vi "Z210 ROUTINE Lister.vi"(0 "unitData in":T3={"typeDevice"=10, "numberDSP"=0}, 2 "DAC#":i32, 3 "buffersParams":T2 {"bufferSize DAC" format="%x"; "bufferAddr DAC" format="%x"; "bufferSize ADC" format="%x"; "bufferAddr ADC" format="%x"}, 5 "error in (no error)":errorcluster, 6 "handicap":dbl=1.0, 7 "Delay Time, ms (100)":i32=-1, 8 "Points":i32, 10 "Linear Correction ADC":T1=[{"scale"=1.0, "offset"=0.0}, {"scale"=1.0, "offset"=0.0}, {"scale"=1.0, "offset"=0.0}, {"scale"=1.0, "offset"=0.0}, {"scale"=1.0, "offset"=0.0}, {"scale"=1.0, "offset"=0.0}, {"scale"=1.0, "offset"=0.0}, {"scale"=1.0, "offset"=0.0}, {"scale"=1.0, "offset"=0.0}, {"scale"=1.0, "offset"=0.0}, {"scale"=1.0, "offset"=0.0}, {"scale"=1.0, "offset"=0.0}, {"scale"=1.0, "offset"=0.0}, {"scale"=1.0, "offset"=0.0}, {"scale"=1.0, "offset"=0.0}, {"scale"=1.0, "offset"=0.0}]) -> (11 "Array":dbl[unit][][](array[numeric]), 14 "unitData out":T3={"typeDevice"=10, "numberDSP"=0}, 17 "buffersParams out":T2 {"bufferSize DAC" format="%x"; "bufferAddr DAC" format="%x"; "bufferSize ADC" format="%x"; "bufferAddr ADC" format="%x"}, 19 "error out":errorcluster)   [LabVIEW 2009]
doc: "Проводится серия следующих измерений: на указанном канале ЦАП устанавливается напряжение в диапазоне 0 - 2,5В (на другом канале ЦАП 0 вольт), затем записываются показания всех каналов АЦП и, если было указано, опрашивается пользователь. Введенное пользователем записывается отдельным каналом в конец.\n\n• unitData — тип устройства и номер сигнального процессора (см. DRIVER Open).\n• AorD — АЦП/ЦАП.\n• numberChannel — номер канала (0 - 16).\n• freq — значение частоты дискретизации в Гц,\n• buffersParams — адреса и размеры буферов данных АЦП и ЦАП в ОЗУ ПК.\n• error in — кластер ошибки. Используется для организации потока данных.\n\n° unitData — тип устройства и номер сигнального процессора (см. DRIVER Open).\n° buffersParams — адреса и размеры буферов данных АЦП и ЦАП в ОЗУ ПК.\n° error out — кластер ошибки. Используется для организации потока данных."
uses:
  Z210/Z210 CTL Lib.llb/Z210 CTL ADC or DAC Function.ctl
  Z210/Z210 CTL Lib.llb/Z210 CTL DAC Voltages.ctl
  Instance          11 27Saved   Z210 ROUTINE Lister .vi
  Z210/Z210 CTL Lib.llb/Z210 CTL Unit Data .ctl
  Z210/Z210 CTL Lib.llb/Z210 CTL Buffers Params.ctl
  Z210/Z210 CTL Lib.llb/Z210 CTL ADC Linear Correction.ctl
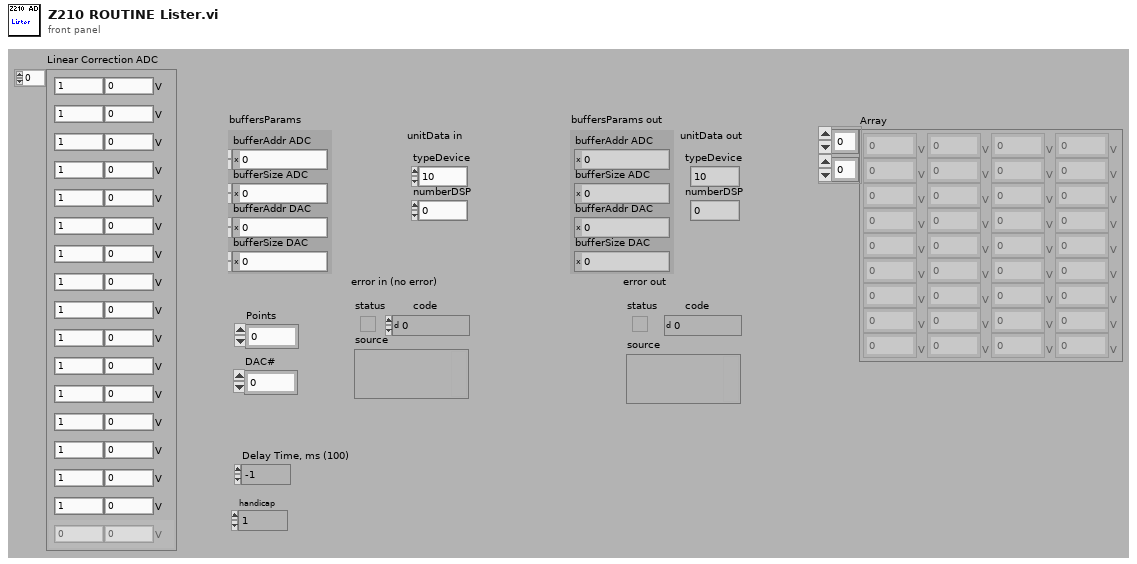
[diagram p1: front panel]
types:
  T1 = typedef "Z210 CTL ADC Linear Correction.ctl" = cluster{"scale":dbl, "offset":dbl[unit]}[]
  T2 = typedef "Z210 CTL Buffers Params.ctl" = cluster{"bufferAddr ADC":u32, "bufferSize ADC":i32, "bufferAddr DAC":u32, "bufferSize DAC":i32}
  T3 = typedef "Z210 CTL Unit Data .ctl" = cluster{"typeDevice":i32, "numberDSP":i32}
  T4 = typedef "Z210 CTL DAC Voltages.ctl" = dbl[unit][]
  T5 = typedef "Z210 CTL ADC or DAC Function.ctl" = enum16{"АЦП", "ЦАП", "Both"}
  T6 = typedef "Z210 CTL ADC Voltages.ctl" = dbl[unit][]
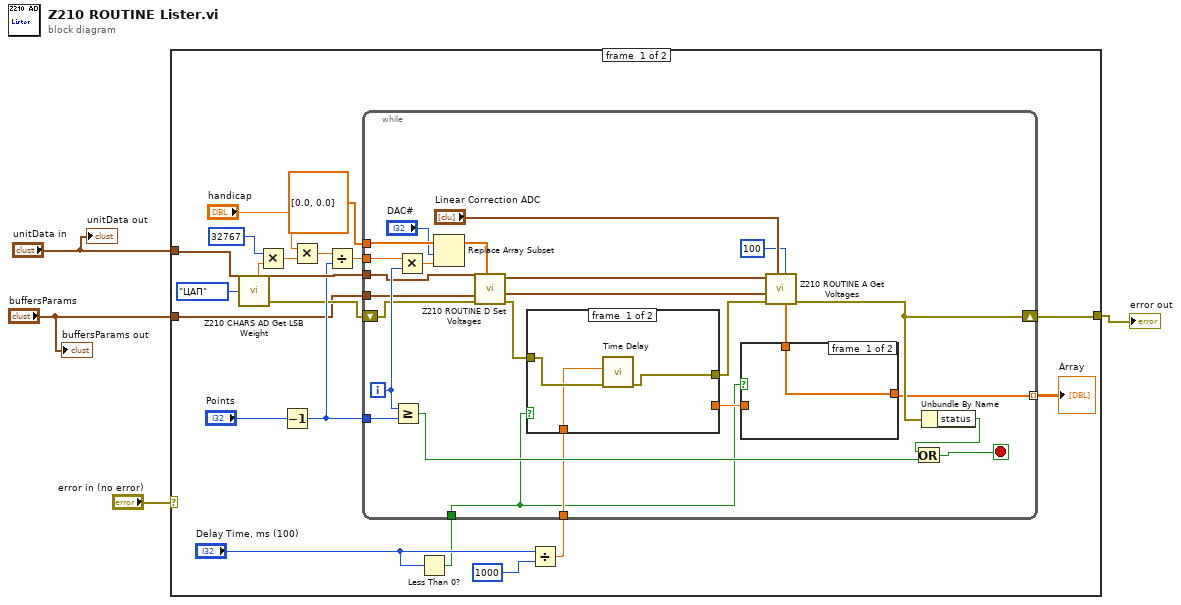
[diagram p0: block diagram]
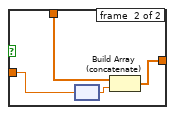
[diagram p2: hidden frame]
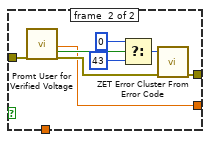
[diagram p3: hidden frame]
diagram:
  n1 = case shown="No Error" "error in (no error)" {
    selector: "error in (no error)" -> [_ w66]
    tunnel: [w12 w66] -> w3
    tunnel: "unitData in" -> [w14 _]
    tunnel: "buffersParams" -> [w13 _]
    frame #0 {
      n2 = call "Z210 CHARS AD Get LSB Weight.vi"("unitData in"=w14, "AorD"=Z210_CTL_ADC_or_DAC_Function."ЦАП") -> ("LBSweight"=w19:dbl[unit], "unitData out"=w24:T3, "error out"=w17:errorcluster)  [unwired: 5 in]
      n3 = Multiply ("Max Volt")(x=i16 32767, y=w19) -> (x*y=w7:dbl[unit])
      n4 = Decrement(x="Points") -> (x-1=w21:i32)
      n5 = Multiply ("Max Volt")(x="handicap", y=w7) -> (x*y=w6:dbl[unit])
      n6 = Divide(x=w6, y=w21) -> (x/y=w22:dbl[unit])
      n7 = Less Than 0?(x="Delay Time, ms (100)") -> (x < 0?=w8:bool)
      n8 = Divide(x="Delay Time, ms (100)", y=1000) -> (x/y=w10:dbl)
      n9 = while {
        tunnel: w21 -> [w49]
        shift-right: [w34] -> w12
        shift-left: w17 -> [w37]
        tunnel: [w31] -> w23 mode=indexing
        tunnel: T4 [0.0, 0.0] ("DAC Voltages") -> [w43]
        tunnel: w22 -> [w42]
        tunnel: w24 -> [w39]
        tunnel: w13 -> [w38]
        tunnel: w10 -> [w26]
        tunnel: w8 -> [w25]
        i -> [w46]
        stop <- w48 stop-if-true
        n10 = Greater Or Equal?(x=w46, y=w49) -> (x >= y?=w47:bool)
        n11 = Multiply(x=w42, y=w46) -> (x*y=w45:dbl[unit])
        n12 = Replace Array Subset(array=w43, new element=w45, index="DAC#") -> (w40:T4)
        n13 = call "Z210 ROUTINE D Set Voltages.vi"("DAC Voltages"=w40, "error in (no error)"=w37, "buffersParams"=w38, "unitData in"=w39) -> ("error out"=w36:errorcluster, "buffersParams out"=w29:T2, "unitData out"=w30:T3)  [unwired: 5 in]
        n14 = case shown="False" w25 {
          tunnel: [w56 w60] -> w35
          tunnel: w36 -> [w57 w59]
          tunnel: [_ w58] -> w33
          tunnel: w26 -> [w55 _]
          frame #0 {
            n15 = call "Time Delay"("error in (no error)"=w57, "Delay Time (s)"=w55) -> ("error out"=w56:errorcluster)  [unwired: 9 in]
          }
          frame #1 {
            n16 = call "Promt User for Verified Voltage.vi"("error in (no error)"=w59) -> ("Verified voltage"=w58:dbl, "OK"=w65:bool, "error out"=w61:errorcluster)  [unwired: 16 in]
            n17 = Select(t=0, s=w65, f=43) -> (s? t:f=w62:i32)
            n18 = call "ZET Error Cluster From Error Code.vi"("error in (no error)"=w61, "error code (0)"=w62) -> ("error out"=w60:errorcluster)  [unwired: 7 in]
          }
        }
        n19 = call "Z210 ROUTINE A Get Voltages.vi"("N to average (1)"=100, "Linear Correction ADC"="Linear Correction ADC", "error in (no error)"=w35, "buffersParams"=w29, "unitData in"=w30) -> ("error out"=w34:errorcluster, "ADC Voltages"=w32:T6)  [unwired: 1 in, 4 out]
        n20 = case shown="True" w25 {
          tunnel: w33 -> [_ w53]
          tunnel: w32 -> [w50 w52]
          tunnel: [w50 w51] -> w31
          frame #0 {
          }
          frame #1 {
            n21 = node(w53) -> (w54:dbl[unit])
            n22 = Build Array (concatenate)(w52, w54) -> (w51:T6)
          }
        }
        n23 = Unbundle By Name(w34) -> ("status"=w44:bool)
        n24 = Or(x=w44, y=w47) -> (x .or. y?=w48:bool)
      }
      "Array" <- w23
    }
    frame #1 {
    }
  }
  "error out" <- w3
  "unitData out" <- "unitData in"
  "buffersParams out" <- "buffersParams"
